vi "预置位巡检.vi"(0 "连接 ID":refnum<k5>, 5 "队列输出":refnum<queue>, 7 "巡检顺序数组":i32[](array[numeric]), 9 "巡检次数":dbl, 11 "到达预置位后等待时间":u32) -> ()   [LabVIEW 2015]
panel:
  out "调用数组":string[](array[string])
  out "过程数组":string[](array[string])
  out "到达数组":string[](array[string])
  out "过程状态":string[](array[string])=["正在去1", "正在去2", "正在去3", "正在去4", "正在去5", "正在去6", "正在去7", "正在去8", "正在去9", "正在去10"]
  out "到达状态":string[](array[string])=["正在去1", "正在去2", "正在去3", "正在去4", "正在去5", "正在去6", "正在去7", "正在去8", "正在去9", "正在去10"]
  out "调用状态":string[](array[string])=["正在去1", "正在去2", "正在去3", "正在去4", "正在去5", "正在去6", "正在去7", "正在去8", "正在去9", "正在去10"]
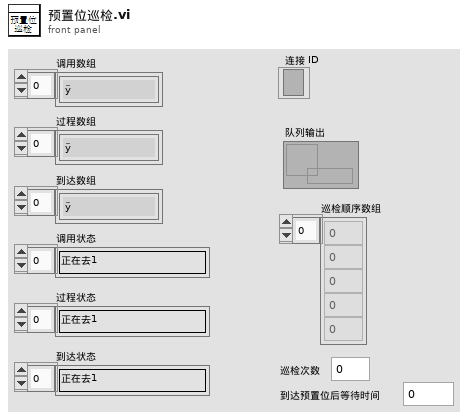
[diagram p1: front panel]
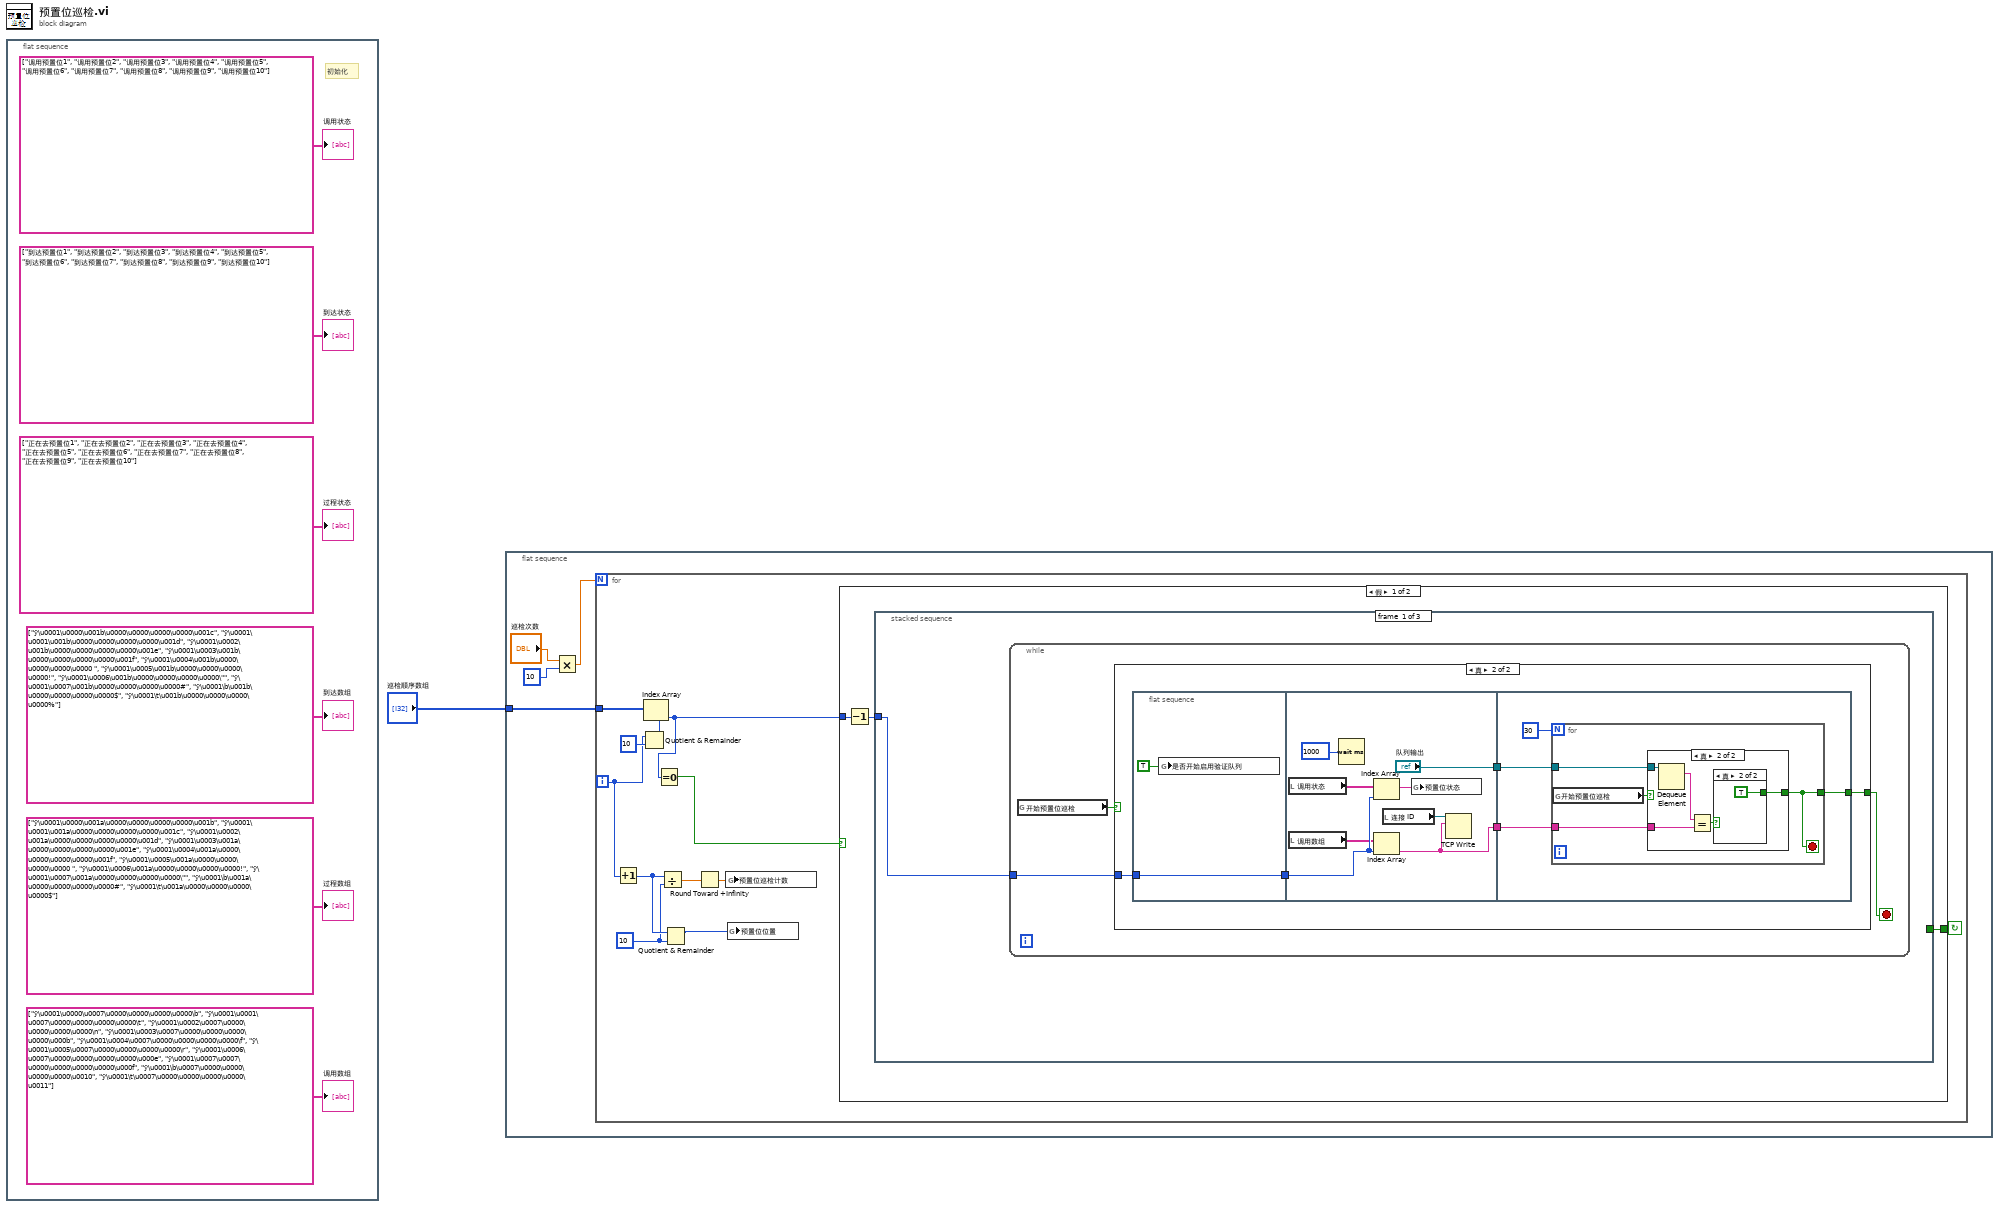
[diagram p0: block diagram]
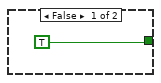
[diagram p2: hidden frame]
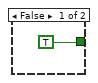
[diagram p3: hidden frame]
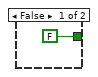
[diagram p4: hidden frame]
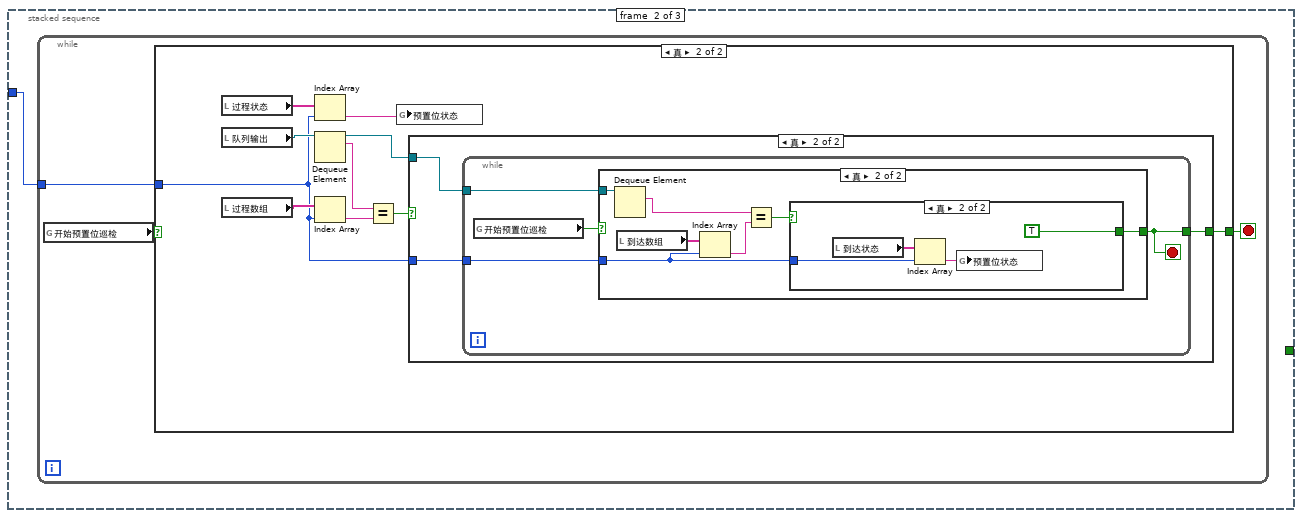
[diagram p5: hidden frame]
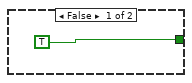
[diagram p6: hidden frame]
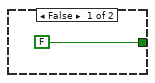
[diagram p7: hidden frame]
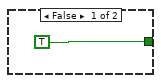
[diagram p8: hidden frame]
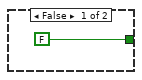
[diagram p9: hidden frame]
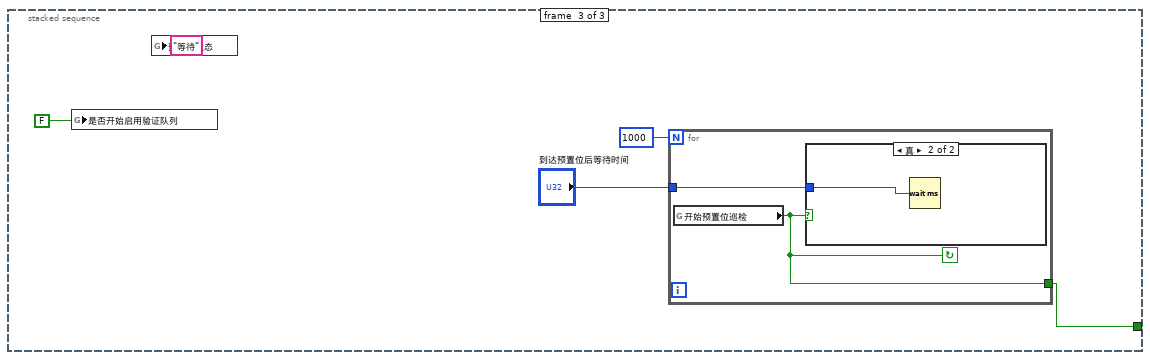
[diagram p10: hidden frame]
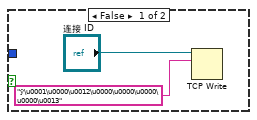
[diagram p11: hidden frame]
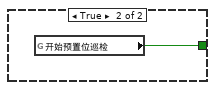
[diagram p12: hidden frame]
diagram:
  n1 = flat-sequence {
    frame #0 {
      # "初始化"
      "调用数组" <- string[] ["ÿ\u0001\u0000\u0007\u0000\u0000\u0000\u0000\b", "ÿ\u0001\u0001\u0007\u0000\u0000\u0000\u0000\t", "ÿ\u0001\u0002\u0007\u0000\u0000\u0000\u0000\n", "ÿ\u0001\u0003\u0007\u0000\u0000\u0000\u0000\u000b", "ÿ\u0001\u0004\u0007\u0000\u0000\u0000\u0000\f", "ÿ\u0001\u0005\u0007\u0000\u0000\u0000\u0000\r", "ÿ\u0001\u0006\u0007\u0000\u0000\u0000\u0000\u000e", "ÿ\u0001\u0007\u0007\u0000\u0000\u0000\u0000\u000f", "ÿ\u0001\b\u0007\u0000\u0000\u0000\u0000\u0010", "ÿ\u0001\t\u0007\u0000\u0000\u0000\u0000\u0011"]
      "过程数组" <- string[] ["ÿ\u0001\u0000\u001a\u0000\u0000\u0000\u0000\u001b", "ÿ\u0001\u0001\u001a\u0000\u0000\u0000\u0000\u001c", "ÿ\u0001\u0002\u001a\u0000\u0000\u0000\u0000\u001d", "ÿ\u0001\u0003\u001a\u0000\u0000\u0000\u0000\u001e", "ÿ\u0001\u0004\u001a\u0000\u0000\u0000\u0000\u001f", "ÿ\u0001\u0005\u001a\u0000\u0000\u0000\u0000 ", "ÿ\u0001\u0006\u001a\u0000\u0000\u0000\u0000!", "ÿ\u0001\u0007\u001a\u0000\u0000\u0000\u0000\"", "ÿ\u0001\b\u001a\u0000\u0000\u0000\u0000#", "ÿ\u0001\t\u001a\u0000\u0000\u0000\u0000$"]
      "到达数组" <- string[] ["ÿ\u0001\u0000\u001b\u0000\u0000\u0000\u0000\u001c", "ÿ\u0001\u0001\u001b\u0000\u0000\u0000\u0000\u001d", "ÿ\u0001\u0002\u001b\u0000\u0000\u0000\u0000\u001e", "ÿ\u0001\u0003\u001b\u0000\u0000\u0000\u0000\u001f", "ÿ\u0001\u0004\u001b\u0000\u0000\u0000\u0000 ", "ÿ\u0001\u0005\u001b\u0000\u0000\u0000\u0000!", "ÿ\u0001\u0006\u001b\u0000\u0000\u0000\u0000\"", "ÿ\u0001\u0007\u001b\u0000\u0000\u0000\u0000#", "ÿ\u0001\b\u001b\u0000\u0000\u0000\u0000$", "ÿ\u0001\t\u001b\u0000\u0000\u0000\u0000%"]
      "过程状态" <- string[] ["正在去预置位1", "正在去预置位2", "正在去预置位3", "正在去预置位4", "正在去预置位5", "正在去预置位6", "正在去预置位7", "正在去预置位8", "正在去预置位9", "正在去预置位10"]
      "到达状态" <- string[] ["到达预置位1", "到达预置位2", "到达预置位3", "到达预置位4", "到达预置位5", "到达预置位6", "到达预置位7", "到达预置位8", "到达预置位9", "到达预置位10"]
      "调用状态" <- string[] ["调用预置位1", "调用预置位2", "调用预置位3", "调用预置位4", "调用预置位5", "调用预置位6", "调用预置位7", "调用预置位8", "调用预置位9", "调用预置位10"]
    }
  }
  n2 = flat-sequence {
    tunnel: "巡检顺序数组" -> [w8]
    frame #0 {
      n3 = Multiply(x="巡检次数", y=10) -> (x*y=w9:dbl)
      n4 = for {
        N: w9 -> [_]
        tunnel: w8 -> [w21]
        i -> [w16]
        stop <- w18 continue-if-true
        w13 = 10
        n5 = Increment(x=w16) -> (x+1=w14:i32)
        n6 = Quotient & Remainder(x=w16, y=10) -> (x-y*floor(x/y)=w22:i32)  [unwired: 1 out]
        n7 = Index Array(array=w21, index=w22) -> (element=w20:i32)
        n8 = Equal To 0?(x=w20) -> (x = 0?=w19:bool)
        n9 = Divide(x=w14, y=w13) -> (x/y=w15:dbl)
        n10 = Quotient & Remainder(x=w14, y=w13) -> (x-y*floor(x/y)=w12:i32)  [unwired: 1 out]
        n11 = Round Toward +Infinity(x=w15) -> (ceil(x): smallest int >= x=w17:dbl)
        n12 = global write "导轨控制全局.vi" "预置位巡检计数"(w17) -> ()
        n13 = global write "导轨控制全局.vi" "预置位位置"(w12) -> ()
        n14 = case shown="假" w19 {
          tunnel: w20 -> [w26 _]
          tunnel: [w24 w109] -> w18
          frame False {
            n15 = Decrement(x=w26) -> (x-1=w25:i32)
            n16 = stacked-sequence {
              tunnel: w25 -> [w27 w63 _]
              tunnel: [_ _ w103] -> w24
              frame #0 {
                n17 = while {
                  tunnel: w27 -> [w30]
                  stop <- w29 stop-if-true
                  n18 = global read "导轨控制全局.vi" "开始预置位巡检"() -> (w28:bool)
                  n19 = case shown="真" w28 {
                    tunnel: w30 -> [_ w33]
                    tunnel: [TRUE w32] -> w29
                    frame False {
                    }
                    frame True {
                      n20 = flat-sequence {
                        tunnel: w33 -> [w38]
                        tunnel: [w38] -> w36
                        tunnel: [w46] -> w35
                        tunnel: ["队列输出"] -> w34
                        tunnel: w36 -> [w43]
                        tunnel: w35 -> [w48]
                        tunnel: w34 -> [w49]
                        tunnel: [w47] -> w32
                        frame #0 {
                          n21 = global write "导轨控制全局.vi" "是否开始启用验证队列"(TRUE) -> ()
                        }
                        frame #1 {
                          n22 = local read "调用状态"() -> (w42:string[])
                          n23 = local read "调用数组"() -> (w41:string[])
                          n24 = Wait (ms)(milliseconds to wait=1000) -> ()  [unwired: 1 out]
                          n25 = Index Array(array=w42, index=w43) -> (element=w40:string)
                          n26 = Index Array(array=w41, index=w43) -> (element=w46:string)
                          n27 = local read "连接 ID"() -> (w45:refnum<k5>)
                          n28 = global write "导轨控制全局.vi" "预置位状态"(w40) -> ()
                          n29 = TCP Write(connection ID=w45, data in=w46) -> ()  [unwired: 2 in, 3 out]
                        }
                        frame #2 {
                          n30 = for {
                            N: 30 -> [_]
                            tunnel: w49 -> [w52]
                            tunnel: [w54] -> w47
                            tunnel: w48 -> [w53]
                            stop <- w54 stop-if-true
                            n31 = global read "导轨控制全局.vi" "开始预置位巡检"() -> (w51:bool)
                            n32 = case shown="真" w51 {
                              tunnel: [TRUE w58] -> w54
                              tunnel: w53 -> [_ w57]
                              tunnel: w52 -> [_ w56]
                              frame False {
                              }
                              frame True {
                                n33 = Dequeue Element(queue=w56) -> (element=w60:string)  [unwired: 2 in, 3 out]
                                n34 = Equal?(x=w60, y=w57) -> (x = y?=w59:bool)
                                n35 = case shown="真" w59 {
                                tunnel: [FALSE TRUE] -> w58
                                frame False {
                                }
                                frame True {
                                }
                                }
                              }
                            }
                          }
                        }
                      }
                    }
                  }
                }
              }
              frame #1 {
                n36 = while {
                  tunnel: w63 -> [w65]
                  stop <- w66 stop-if-true
                  n37 = global read "导轨控制全局.vi" "开始预置位巡检"() -> (w64:bool)
                  n38 = case shown="真" w64 {
                    tunnel: [TRUE w71] -> w66
                    tunnel: w65 -> [_ w70]
                    frame False {
                    }
                    frame True {
                      n39 = local read "过程状态"() -> (w69:string[])
                      n40 = local read "队列输出"() -> (w75:refnum<queue>)
                      n41 = local read "过程数组"() -> (w74:string[])
                      n42 = Index Array(array=w69, index=w70) -> (element=w68:string)
                      n43 = Dequeue Element(queue=w75) -> (queue out=w72:refnum<queue>, element=w77:string)  [unwired: 2 in, 2 out]
                      n44 = Index Array(array=w74, index=w70) -> (element=w73:string)
                      n45 = Equal?(x=w77, y=w73) -> (x = y?=w76:bool)
                      n46 = global write "导轨控制全局.vi" "预置位状态"(w68) -> ()
                      n47 = case shown="真" w76 {
                        tunnel: w72 -> [_ w81]
                        tunnel: [FALSE w80] -> w71
                        tunnel: w70 -> [_ w79]
                        frame False {
                        }
                        frame True {
                          n48 = while {
                            tunnel: w81 -> [w85]
                            tunnel: [w83] -> w80
                            tunnel: w79 -> [w84]
                            stop <- w83 stop-if-true
                            n49 = global read "导轨控制全局.vi" "开始预置位巡检"() -> (w82:bool)
                            n50 = case shown="真" w82 {
                              tunnel: w85 -> [_ w93]
                              tunnel: w84 -> [_ w88]
                              tunnel: [TRUE w87] -> w83
                              frame False {
                              }
                              frame True {
                                n51 = Dequeue Element(queue=w93) -> (element=w91:string)  [unwired: 2 in, 3 out]
                                n52 = local read "到达数组"() -> (w92:string[])
                                n53 = Index Array(array=w92, index=w88) -> (element=w90:string)
                                n54 = Equal?(x=w91, y=w90) -> (x = y?=w89:bool)
                                n55 = case shown="真" w89 {
                                tunnel: [FALSE TRUE] -> w87
                                tunnel: w88 -> [_ w96]
                                frame False {
                                }
                                frame True {
                                n56 = local read "到达状态"() -> (w97:string[])
                                n57 = Index Array(array=w97, index=w96) -> (element=w95:string)
                                n58 = global write "导轨控制全局.vi" "预置位状态"(w95) -> ()
                                }
                                }
                              }
                            }
                          }
                        }
                      }
                    }
                  }
                }
              }
              frame #2 {
                n59 = global write "导轨控制全局.vi" "是否开始启用验证队列"(FALSE) -> ()
                n60 = global write "导轨控制全局.vi" "预置位状态"("等待") -> ()
                n61 = for {
                  N: 1000 -> [_]
                  tunnel: "到达预置位后等待时间" -> [w105]
                  tunnel: [w104] -> w103
                  stop <- w104 continue-if-true
                  n62 = global read "导轨控制全局.vi" "开始预置位巡检"() -> (w104:bool)
                  n63 = case shown="真" w104 {
                    tunnel: w105 -> [_ w108]
                    frame False {
                      n64 = TCP Write(connection ID="连接 ID", data in="ÿ\u0001\u0000\u0012\u0000\u0000\u0000\u0000\u0013") -> ()  [unwired: 2 in, 3 out]
                    }
                    frame True {
                      n65 = Wait (ms)(milliseconds to wait=w108) -> ()  [unwired: 1 out]
                    }
                  }
                }
              }
            }
          }
          frame True {
            n66 = global read "导轨控制全局.vi" "开始预置位巡检"() -> (w109:bool)
          }
        }
      }
    }
  }
